vi "RM-read-current-position.vi"(8 "错误输入（无错误）":errorcluster, 11 "MB_Master_Serial输入":refnum<class "MB_Master_Serial.lvclass">) -> (0 "错误输出":errorcluster, 2 "数值":dbl, 3 "MB_Master_Serial输出":refnum<class "MB_Master_Serial.lvclass">)   [LabVIEW 2014]
uses:
  <vilib>/Plasmionique/MB Master/MB_Master_Serial/MB_Master_Serial.lvclass
  <vilib>/Plasmionique/MB Master/MB Master.lvlib
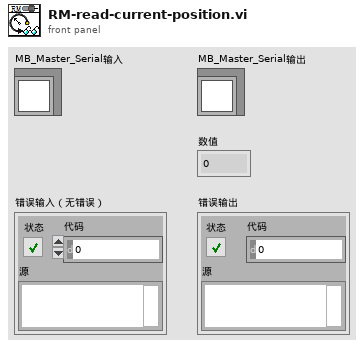
[diagram p1: front panel]
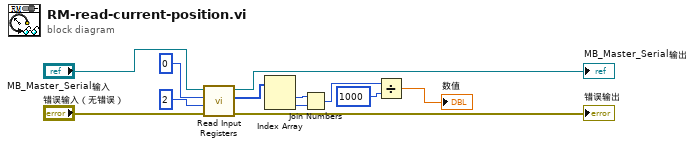
[diagram p0: block diagram]
diagram:
  n1 = call <vilib>:"Read Input Registers.vi"("error in (no error)"="错误输入（无错误）", "quantity"=u16 2, "starting address"=u16 0, "MB session in"="MB_Master_Serial输入") -> ("error out"=→"错误输出":errorcluster, "Registers"=w7:u16[], "MB session out"=→"MB_Master_Serial输出":refnum<class "MB_Master_Serial.lvclass">)  [unwired: 5 in]
  n2 = Index Array(array=w7) -> (element #1=w8:u16, element #2=w9:u16)  [unwired: 2 in]
  n3 = Join Numbers(hi=w8, lo=w9) -> ((hi.lo)=w10:u32)
  n4 = Divide(x=w10, y=u32 1000) -> (x/y=→"数值":dbl)
